vi "XIPIN_Video_Test_Pattern_Generator_7_0.vi"   [LabVIEW 2017]
doc: "The Xilinx Video Test Pattern Generator creates test-patterns that are useful in the development of video IP blocks. The patterns may also be used in-system for display purposes.\n------------------------------------\n<b>Need License</b> : Yes\n<b>Interface</b> : AXI4 AXI4-Stream"
uses:
  <vilib>/rvi/XilinxIP/XIPIN_XNode/niFpgaXIPIN.xnode
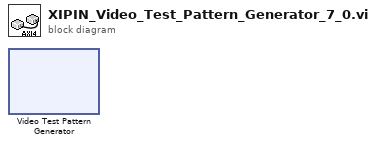
[diagram p0: block diagram]
diagram:
  n1 = xnode ("Video Test Pattern Generator")() -> ()
